vi "Handle TCP Message.vi"(7 "TCPMessageAPI":refnum<class "TCPMessageAPI.lvclass">, 8 "error in (no error)":errorcluster, 10 "TcpPayload":T1, 11 "RemoteMessagingHandler in":refnum<class "RemoteMessagingHandler.lvclass">) -> (0 "error out":errorcluster, 3 "RemoteMessagingHandler out":refnum<class "RemoteMessagingHandler.lvclass">)   [LabVIEW 2020, in "Volatus.lvlib" / "RemoteMessagingHandler.lvclass"]
uses:
  RemoteMessagingHandler.lvclass
  lv-vecto/Vecto/TCPMessageService/TCPMessageAPI.lvclass
  lv-vecto/Vecto/proto/TcpPayload/Data.ctl
  RemoteMessagingHandler.lvclass/RemoteMessagingHandler.ctl
  RemoteMessaging Messages/New Message Msg/New Message Msg.lvclass
  lv-vecto/Vecto/proto/TcpPayload/TcpPayload.lvlib
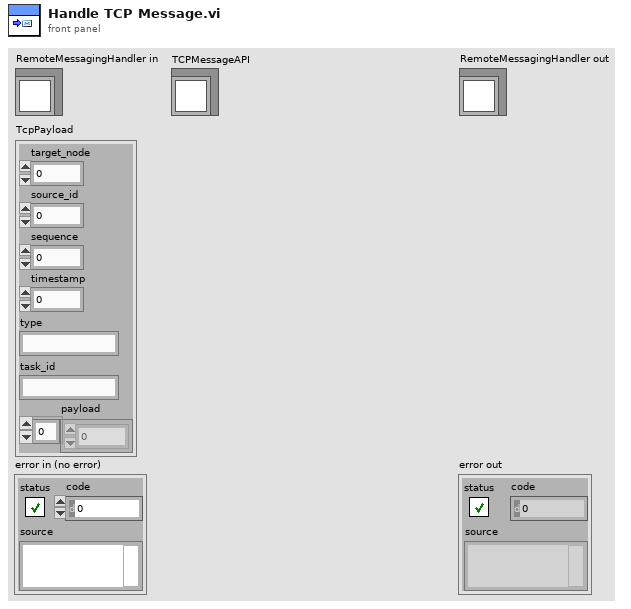
[diagram p1: front panel]
types:
  T1 = typedef "TcpPayload.lvlib/Data.ctl" = cluster{"target_node":u32, "source_id":u32, "sequence":u32, "timestamp":u64, "type":string, "task_id":string, "payload":u8[]}
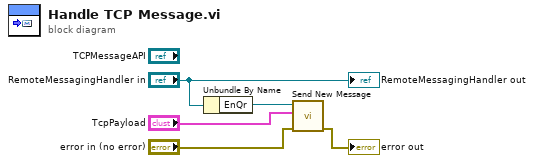
[diagram p0: block diagram]
diagram:
  n1 = Unbundle By Name("RemoteMessagingHandler in") -> ("EnQr"=w4:refnum<class "Message Enqueuer.lvclass">)
  n2 = call "Send New Message.vi"("error in (no error)"="error in (no error)", "TcpPayload"="TcpPayload", "Message Enqueuer"=w4) -> ("error out"=→"error out":errorcluster)  [unwired: 7 in, 1 out]
  "RemoteMessagingHandler out" <- "RemoteMessagingHandler in"
